vi "Convert activity log to string table.vi"(3 "Chars per line":u8, 4 "Activity Array":T1(array[cluster])) -> (1 "Table":string[][](table))   [LabVIEW 2009]
doc: "Converts the activity array into a 2-D string table for viewing in a table. Chars per line determines how many characters should go in each line of the activity (a manual word wrap feature). \n\nACTIVTY ARRAY IN IS REVERSED SO MOST RECENT ACTIVITY IOS FIRST!"
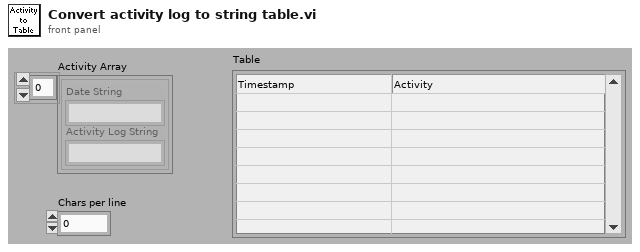
[diagram p1: front panel]
types:
  T1 = cluster{"Date String":string, "Activity Log String":string}[]
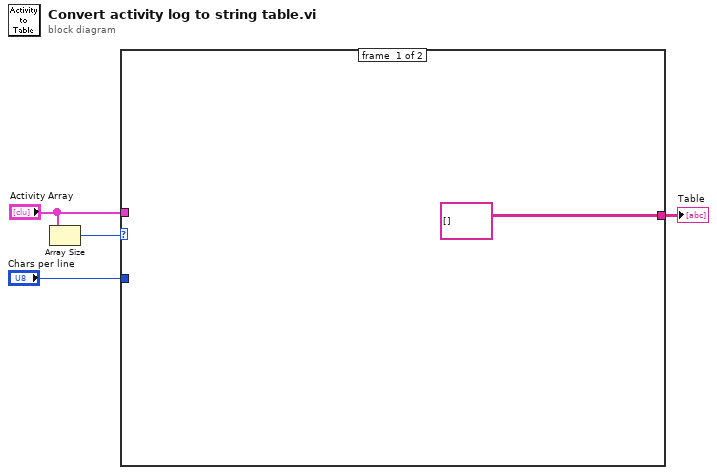
[diagram p0: block diagram]
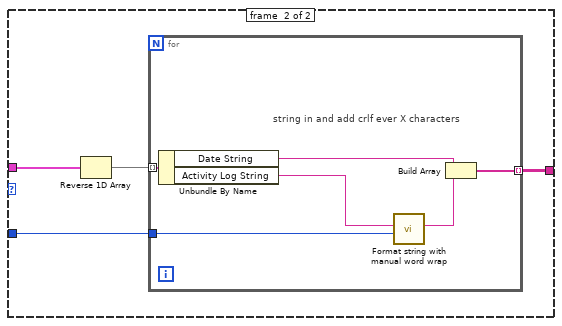
[diagram p2: hidden frame]
diagram:
  n1 = Array Size(array="Activity Array") -> (size(s)=w4:i32)
  n2 = case shown="1, Default" w4 {
    tunnel: "Activity Array" -> [_ w7]
    tunnel: [string[][] [] w9] -> w3
    tunnel: "Chars per line" -> [_ w8]
    frame #0 {
    }
    frame #1 {
      n3 = Reverse 1D Array(array=w7) -> (reversed array=w6:T1)
      n4 = for {
        tunnel: w6 -> [w15] mode=indexing
        tunnel: [w14] -> w9 mode=indexing
        tunnel: w8 -> [w11]
        # "string in and add crlf ever X characters"
        n5 = Unbundle By Name(w15) -> ("Date String"=w13:string, "Activity Log String"=w12:string)
        n6 = call "Format string with manual word wrap .vi"("Chars per line"=w11, "String"=w12) -> ("String with manual Word Wrap"=w10:string)  [unwired: 5 out]
        n7 = Build Array(w13, w10) -> (w14:string[])
      }
    }
  }
  "Table" <- w3
